vi "Execute.vi"(8 "error in (no error)":errorcluster, 10 "Abstract Consumer in":refnum<class "Abstract Consumer.lvclass">, 11 "Log Word Message in":refnum<class "Log Message.lvclass">) -> (0 "error out":errorcluster, 1 "Abstract Response out":refnum<class "Abstract Response Message.lvclass">, 2 "Abstract Consumer out":refnum<class "Abstract Consumer.lvclass">, 3 "Log Word Message out":refnum<class "Log Message.lvclass">, 4 "Stop?":bool)   [LabVIEW 2020, in "AIM MIL-STD-1553 Engine.lvlib" / "Implementation.lvlib" / "Word Logging.lvlib" / "Log Message.lvclass"]
uses:
  Log Message.lvclass
  <vilib>/NI/VeriStand Custom Device Messaging/Consumer/Abstract Consumer/Abstract Consumer.lvclass
  <vilib>/NI/VeriStand Custom Device Messaging/Message/Abstract Response Message/Abstract Response Message.lvclass
  Logger Interface/Logger Interface.lvclass
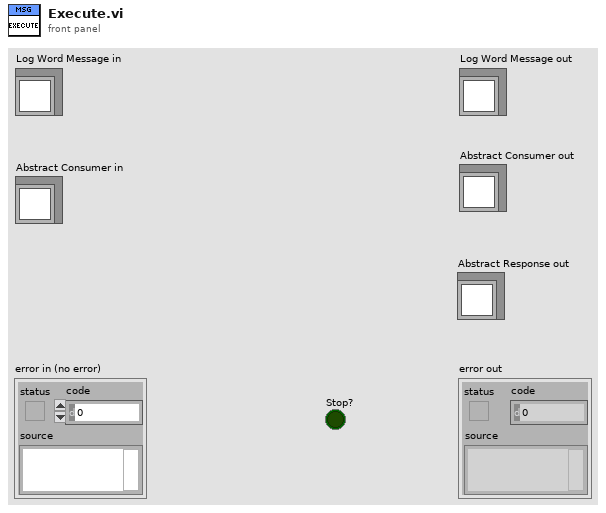
[diagram p1: front panel]
types:
  T1 = typedef "AIM MIL-STD-1553 Engine.lvlib/Implementation.lvlib/Word Logging.lvlib/Logger Data Reference.ctl" = refnum<data-value>
  T2 = typedef "Log Entry.ctl" = cluster{"Queue Entry":T3, "Message Data Buffer":u16[]}
  T3 = typedef "1553 BM Queue Entry.ctl" = cluster{"RT Address":u8, "Sub-address":u8, "Mode Code":enum16{"Dynamic bus control", "Synchronize", "Transmit status word", "Initiate self test", "Transmitter shutdown", "Override transmitter shutdown", "Inhibit terminal flag bit", "Override inhibit terminal flag bit", "Reset remote terminal", "(reserved)", "(reserved) ", "(reserved)  ", "(reserved)   ", "(reserved)    ", "(reserved)     ", "(reserved)      ", "Transmit vector word", "Synchronize ", "Transmit last command", "Transmit bit word", "Selected xmtr shutdown", "Override selected xmtr shutdown", "(reserved)       ", "(reserved)        ", "(reserved)         ", "(reserved)          ", "(reserved)           ", "(reserved)            ", "(reserved)             ", "(reserved)              ", "(reserved)               ", "(reserved)                "}, "Direction":enum16{"receive", "transmit"}, "Type":enum16{"sub-address", "mode code"}, "RT Address 2":u8, "Sub-address 2":u8, "Mode Code 2":enum16{"Dynamic bus control", "Synchronize", "Transmit status word", "Initiate self test", "Transmitter shutdown", "Override transmitter shutdown", "Inhibit terminal flag bit", "Override inhibit terminal flag bit", "Reset remote terminal", "(reserved)", "(reserved) ", "(reserved)  ", "(reserved)   ", "(reserved)    ", "(reserved)     ", "(reserved)      ", "Transmit vector word", "Synchronize ", "Transmit last command", "Transmit bit word", "Selected xmtr shutdown", "Override selected xmtr shutdown", "(reserved)       ", "(reserved)        ", "(reserved)         ", "(reserved)          ", "(reserved)           ", "(reserved)            ", "(reserved)             ", "(reserved)              ", "(reserved)               ", "(reserved)                "}, "Direction 2":enum16{"receive", "transmit"}, "Type 2":enum16{"sub-address", "mode code"}, "Word Count":u8, "Bus":enum16{"primary", "secondary"}, "Minutes":i32, "Seconds":i32, "Microseconds":i32, "Error ":enum16{"No error", "Terminal no response error", "Manchester coding error", "High bit count error", "Low bit count error", "Parity error", "Inverted sync error", "Interw ord gap error", "Transmission on both MILbus channels", "Reserved mode code error", "Early response or gap too short", "ME bit set in status word", "Status word exception error", "High wordcount error", "Low wordcount error", "Illegal command word"}}
  T4 = cluster{"Logger Interface":refnum<class "Logger Interface.lvclass">}
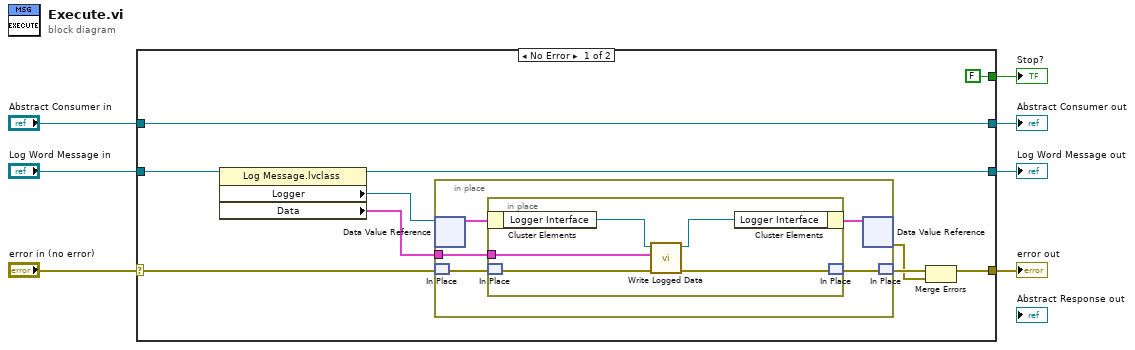
[diagram p0: block diagram]
diagram:
  n1 = case shown="No Error" "error in (no error)" {
    selector: "error in (no error)" -> [w13 w30]
    tunnel: [w10 w30] -> w6
    tunnel: [w17 w28] -> w5
    tunnel: "Abstract Consumer in" -> [w17 w28]
    tunnel: [FALSE ("Stop?") _] -> w3
    tunnel: [w14 w29] -> w2
    tunnel: "Log Word Message in" -> [w15 w29]
    frame No Error {
      n2 = property class="Log Message.lvclass"(reference=w15) -> (reference out=w14:refnum<class "Log Message.lvclass">, "Logger"=w11:T1, "Data"=w8:T2[])  [unwired: 1 in, 1 out]
      n3 = in-place {
        in-place-border: w8 -> [w22]
        n4 = in-place-dvr #1(w11) -> (w19:T4)  [unwired: 1 out]
        n5 = in-place-match #2(w13) -> (w21:errorcluster)
        n6 = in-place {
          in-place-border: w22 -> [w23]
          n7 = in-place-cluster #3(w19) -> ("Logger Interface"=w25:refnum<class "Logger Interface.lvclass">)
          n8 = in-place-match #4(w21) -> (w27:errorcluster)
          n9 = call-dynamic "Write Logged Data.vi"("error in (no error)"=w27, "Data"=w23, "Logger Interface in"=w25) -> ("error out"=w26:errorcluster, "Logger Interface out"=w24:refnum<class "Logger Interface.lvclass">)  [unwired: 7 in]
          n10 = in-place-cluster #3("Logger Interface"=w24) -> (w18:T4)
          n11 = in-place-match #4(w26) -> (w20:errorcluster)
        }
        n12 = in-place-dvr #1(w18) -> (w9:errorcluster)  [unwired: 1 out]
        n13 = in-place-match #2(w20) -> (w12:errorcluster)
      }
      n14 = Merge Errors(w12, w9) -> (w10:errorcluster)
    }
    frame Error {
    }
  }
  "error out" <- w6
  "Log Word Message out" <- w2
  "Abstract Consumer out" <- w5
  "Stop?" <- w3
